vi "Panel.vi"(11 "Battery Stack in":refnum<class "Battery Stack.lvclass">) -> ()   [LabVIEW 2020, in "Battery Stack.lvclass"]
uses:
  Battery Stack.lvclass
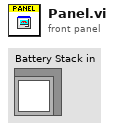
[diagram p1: front panel]
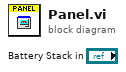
[diagram p0: block diagram]
diagram:
